vi "Wait for Samples Ready.vi"(5 "timeout in milliseconds":u32=5000, 8 "error in (no error)":errorcluster, 9 "minimum ready samples":u32, 10 "stream index":i32, 11 "refnum in":refnum<k20>) -> (0 "error out":errorcluster, 1 "samples ready":u32, 3 "refnum out":refnum<k20>)   [LabVIEW 2015, in "niInstr Streaming v1 Host.lvlib"]
doc: "Waits until the number of requested samples report that they are ready. This corresponds to the Monitor FIFO Health.vi output - stream.num samples ready (N), where (N) corresponds to the <b>stream index</b> input.\n\nIf the stream is unable to prime to this level within the time specified, a timeout error is reported.\n\n<B>Input Parameters</B>\n\n<B>timeout in milliseconds</B> Maximum time to wait for the stream to report 'stream.num samples ready' >= 'minimum ready samples'\n\n<B>error in (no error)</B> 'error in' can accept error information wired from VIs previously called. Use this information to decide if any functionality should be bypassed in the event of errors from other VIs.\n\nRight-click the 'error in' control on the front panel and select 'Explain Error' or 'Explain Warning' from the shortcut menu for more information about the error.\n\n<B>stream index</B> Selects which stream index this VI will interface to. This is the index number at the end of the host interface controls (0..7).\n\n<B>refnum in</B> Wire in the session obtained from Open FPGA Reference.\n\n<B>Output Parameters</B>\n\n<B>error out</B> contains error information. This output provides standard error out functionality.\n\n<B>refnum out</B> Copy of refnum in"
uses:
  <instrlib>/_niInstr/Streaming/v1/Host/niInstr Streaming v1 Host.lvlib
  <vilib>/Utility/error.llb/Error Cluster From Error Code.vi
  <vilib>/ErrorRing/Error Ring.xnode
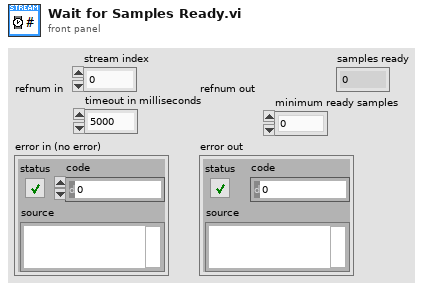
[diagram p1: front panel]
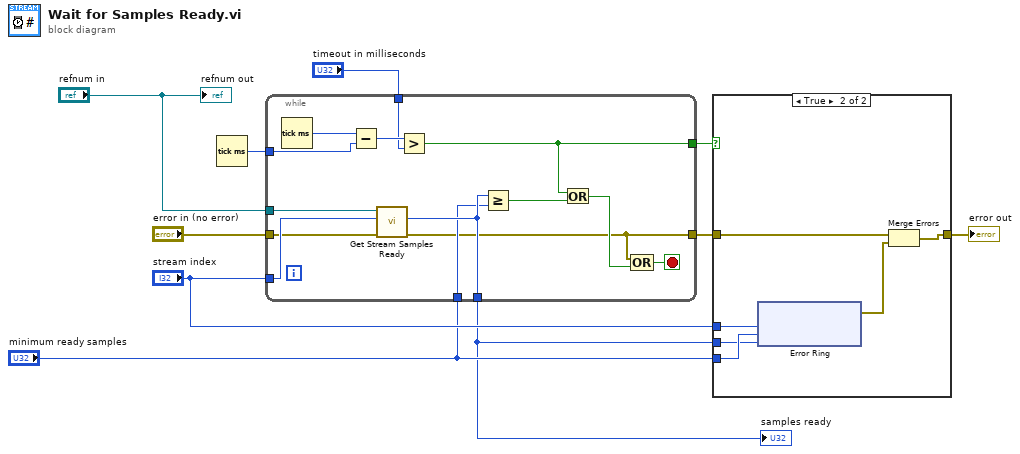
[diagram p0: block diagram]
diagram:
  n1 = Tick Count (ms)() -> (millisecond timer value=w10:u32)
  n2 = while {
    tunnel: "refnum in" -> [w12]
    tunnel: "error in (no error)" -> [w13]
    tunnel: w10 -> [w23]
    tunnel: [w11] -> w5
    tunnel: [w20] -> w1
    tunnel: "stream index" -> [w18]
    tunnel: "timeout in milliseconds" -> [w19]
    tunnel: "minimum ready samples" -> [w16]
    tunnel: [w17] -> w2
    stop <- w24 stop-if-true
    n3 = Tick Count (ms)() -> (millisecond timer value=w22:u32)
    n4 = Subtract(x=w22, y=w23) -> (x-y=w21:u32)
    n5 = call <instrlib>:"Get Stream Samples Ready.vi"("error in (no error)"=w13, "stream index"=w18, "refnum in"=w12) -> ("error out"=w11:errorcluster, "samples ready"=w17:u32)  [unwired: 6 in, 1 out]
    n6 = Greater?(x=w21, y=w19) -> (0:w20:bool)
    n7 = Greater Or Equal?(x=w17, y=w16) -> (x >= y?=w14:bool)
    n8 = Or(x=w20, y=w14) -> (x .or. y?=w15:bool)
    n9 = Compound Arithmetic op=OR(w11, w15) -> (w24:bool)
  }
  "samples ready" <- w2
  n10 = case shown="True" w1 {
    tunnel: [w25 w31] -> w6
    tunnel: w5 -> [w25 w30]
    tunnel: "stream index" -> [_ w28]
    tunnel: "minimum ready samples" -> [_ w27]
    tunnel: w2 -> [_ w26]
    frame False {
    }
    frame True {
      n11 = xnode "Error Ring"("parameter 0"=w28, "parameter 1"=w27, "parameter 2"=w26) -> ("error out"=w29:errorcluster)
      n12 = Merge Errors(w30, w29) -> (w31:errorcluster)
    }
  }
  "error out" <- w6
  "refnum out" <- "refnum in"
